vi "Simple TCP Client.vi"() -> ()   [LabVIEW 2023, in "VectoScratch.lvlib"]
uses:
  VectoScratch.lvlib
  Vecto/Connection State.ctl
  Vecto/proto/ConstellationCommand/Data.ctl
  Vecto/proto/TcpClientHello/Data.ctl
  Constellation Command Handler/Constellation Command Handler.lvclass/Constellation Command Handler.ctl
  Constellation Command Handler/Constellation Command Handler.lvclass
  C:/Users/zcoll/Documents/constellation/lv-vecto/Vecto/TCPMessageHandler/TCPMessageHandler.lvclass
  C:/Users/zcoll/Documents/constellation/lv-vecto/Vecto/TCPConnectionHandler/TCPConnectionHandler.lvclass
  Vecto/SequenceCountService/SequenceCountService.lvclass
  Vecto/TCPMessaging/TCPMessaging.lvclass
  Vecto/proto/TcpClientHello/TcpClientHello.lvlib
  Vecto/TCPMessageService/TCPMessageAPI.lvclass
  Vecto/proto/ConstellationCommand/ConstellationCommand.lvlib
  Vecto/Vecto.lvlib
panel:
  out "Command":T1 {"Time Stamp" format="%<%x %.3X>T"}
  out "error out":errorcluster
  in  "Client Stop":bool
  out "Client State":T2=enum."Disconnected"
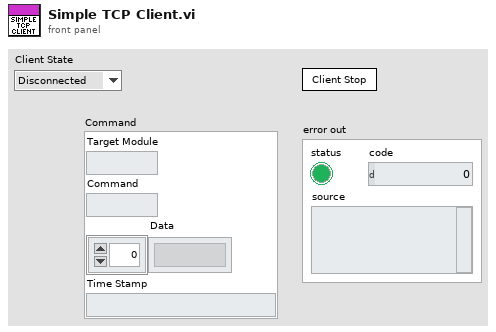
[diagram p1: front panel]
types:
  T1 = typedef "ConstellationCommand.lvlib/Data.ctl" = cluster{"Target Module":string, "Command":string, "Data":string[], "Time Stamp":timestamp}
  T2 = typedef "Vecto.lvlib/Connection State.ctl" = enum16{"Connected", "Disconnected"}
  T3 = typedef "TcpClientHello.lvlib/Data.ctl" = cluster{"node_id":u32, "system":string, "cluster":string, "node_name":string, "app_version":string, "config_version":string}
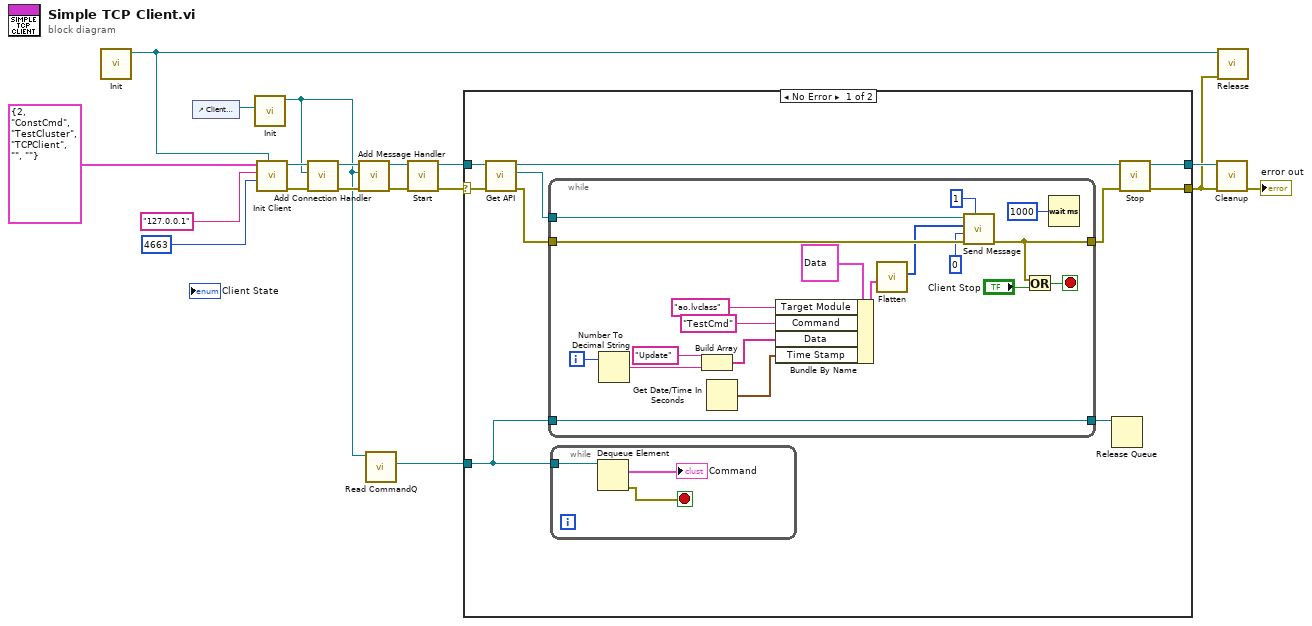
[diagram p0: block diagram]
diagram:
  n1 = call "Init.vi"() -> ("SequenceCountService out"=w14:refnum<class "SequenceCountService.lvclass">)  [unwired: 10 in, 1 out]
  n2 = control-ref of="Client State"() -> (w3:refnum<vi>)
  n3 = call "Init.vi"("State"=w3) -> ("Constellation Command Handler out"=w2:refnum<class "Constellation Command Handler.lvclass">)  [unwired: 10 in]
  n4 = call "Init Client.vi"("SequenceCountService"=w14, "Remote Port"=u16 4663, "Remote Address"="127.0.0.1", "Client Info"=T3 {"node_id"=2, "system"="ConstCmd", "cluster"="TestCluster", "node_name"="TCPClient", "app_version"="", "config_version"=""}) -> ("error out"=w9:errorcluster, "TCPMessaging out"=w16:refnum<class "TCPMessaging.lvclass">)  [unwired: 6 in]
  n5 = call "Add Connection Handler.vi"("error in (no error)"=w9, "TCPConnectionHandler"=w2, "TCPMessaging in"=w16) -> ("error out"=w8:errorcluster, "TCPMessaging out"=w17:refnum<class "TCPMessaging.lvclass">)  [unwired: 7 in]
  n6 = call "Add Message Handler.vi"("error in (no error)"=w8, "TCPMessageHandler"=w2, "TCPMessaging in"=w17) -> ("error out"=w7:errorcluster, "TCPMessaging out"=w18:refnum<class "TCPMessaging.lvclass">)  [unwired: 7 in]
  n7 = call "Read CommandQ.vi"("Constellation Command Handler in"=w2) -> ("CommandQ"=w1:refnum<queue>)  [unwired: 9 in, 1 out]
  n8 = call "Start.vi"("error in (no error)"=w7, "TCPMessaging in"=w18) -> ("error out"=w13:errorcluster, "TCPMessaging out"=w12:refnum<class "TCPMessaging.lvclass">)  [unwired: 8 in]
  n9 = case shown="No Error" w13 {
    selector: w13 -> [w27 w51]
    tunnel: w12 -> [w28 w52]
    tunnel: [w23 w52] -> w11
    tunnel: [w21 w51] -> w10
    tunnel: w1 -> [w20 _]
    frame No Error {
      n10 = call "Get API.vi"("error in (no error)"=w27, "TCPMessaging in"=w28) -> ("error out"=w25:errorcluster, "TCP Messaging API"=w26:refnum<class "TCPMessageAPI.lvclass">, "TCPMessaging out"=w24:refnum<class "TCPMessaging.lvclass">)  [unwired: 7 in]
      n11 = while {
        tunnel: w26 -> [w50]
        tunnel: w25 -> [w48]
        tunnel: [w43] -> w22
        tunnel: w20 -> [w32]
        tunnel: [w32] -> w19
        i -> [w37]
        stop <- w44 stop-if-true
        n12 = Number To Decimal String(number=w37) -> (decimal integer string=w36:string)  [unwired: 1 in]
        n13 = Build Array("Update" ("Command"), w36) -> (w39:string[])
        n14 = Get Date/Time In Seconds() -> (seconds since 1Jan1904=w34:timestamp)
        n15 = Bundle By Name(cluster=T1 {"Target Module"="", "Command"="", "Data"=[], "Time Stamp"=timestamp(0 s since 1904-01-01)} ("Command Data"), "Target Module"="ao.lvclass", "Command"="TestCmd", "Data"=w39, "Time Stamp"=w34) -> (w33:T1)
        n16 = call "Flatten.vi"("Command Data"=w33) -> ("Buffer"=w42:u8[])  [unwired: 9 in, 1 out]
        n17 = call "Send Message.vi"("Target Node"=u32 1, "error in (no error)"=w48, "Type ID"=u32 0, "Payload"=w42, "TCPMessageService in"=w50) -> ("error out"=w43:errorcluster)  [unwired: 5 in, 1 out]
        n18 = Or(x=w43, y="Client Stop") -> (x .or. y?=w44:bool)
        n19 = Wait (ms)(milliseconds to wait=u32 1000) -> ()  [unwired: 1 out]
      }
      n20 = while {
        tunnel: w20 -> [w31]
        stop <- w29 stop-if-true
        n21 = Dequeue Element(queue=w31) -> (element=→"Command":T1, error out=w29:errorcluster)  [unwired: 2 in, 2 out]
      }
      n22 = Release Queue(queue=w19) -> ()  [unwired: 2 in, 3 out]
      n23 = call "Stop.vi"("error in (no error)"=w22, "TCPMessaging in"=w24) -> ("error out"=w21:errorcluster, "TCPMessaging out"=w23:refnum<class "TCPMessaging.lvclass">)  [unwired: 8 in]
    }
    frame Error {
    }
  }
  n24 = call "Cleanup.vi"("error in (no error)"=w10, "TCPMessaging in"=w11) -> ("error out"=→"error out":errorcluster)  [unwired: 9 in]
  n25 = call "Release.vi"("error in (no error)"=w10, "SequenceCountService in"=w14) -> ()  [unwired: 9 in, 1 out]
